vi "OpenCloseThreadWin.vi"(0 "reference in":refnum<class "SuperNS.lvclass">, 2 "Open (F: Close)":bool, 5 "error in":errorcluster) -> (14 "reference out":refnum<class "SuperNS.lvclass">, 19 "error out":errorcluster)   [LabVIEW 2020, in "SuperNS.lvclass"]
doc: "Copyright © 2008 - 2024 VI Technologies B.V. \nALL RIGHTS RESERVED\n\nOpens / Closes the SuperNS's background process frontpanel. This could be usefull for debugging purposes."
uses:
  SuperNS.lvclass
  SuperNS.lvclass/SuperNS.ctl
panel:
  # "Copyright (c) 2024, VI Technologies B.V.\nAll rights reserved.\n\nRedistribution and use in source and binary forms, with or without modification, are permitted provided that \nthe following conditions are met:\n\n * Redistributions of source code must retain the above copyright notice, this list of conditions and the \nfollowing disclaimer.\n * Redistributions in binary form must reproduce the above copyright notice, this list of conditions and the \nfollowing disclaimer in the documentation and/or other materials provided with the distribution.\n * Neither the name of VI Technologies B.V. nor the names of its contributors may be used to endorse or \npromote products derived from this software without specific prior written permission.\n\nTHIS SOFTWARE IS PROVIDED BY THE COPYRIGHT HOLDERS AND CONTRIBUTORS \"AS IS\" AND ANY EXPRESS OR \nIMPLIED WARRANTIES, INCLUDING, BUT NOT LIMITED TO, THE IMPLIED WARRANTIES OF MERCHANTABILITY \nAND FITNESS FOR A PARTICULAR PURPOSE ARE DISCLAIMED. IN NO EVENT SHALL THE COPYRIGHT OWNER OR \nCONTRIBUTORS BE LIABLE FOR ANY DIRECT, INDIRECT, INCIDENTAL, SPECIAL, EXEMPLARY, OR CONSEQUENTIAL \nDAMAGES (INCLUDING, BUT NOT LIMITED TO, PROCUREMENT OF SUBSTITUTE GOODS OR SERVICES; LOSS OF \nUSE, DATA, OR PROFITS; OR BUSINESS INTERRUPTION) HOWEVER CAUSED AND ON ANY THEORY OF LIABILITY, \nWHETHER IN CONTRACT, STRICT LIABILITY, OR TORT (INCLUDING NEGLIGENCE OR OTHERWISE) ARISING IN ANY \nWAY OUT OF THE USE OF THIS SOFTWARE, EVEN IF ADVISED OF THE POSSIBILITY OF SUCH DAMAGE.\n\nFor more information, please visit https://www.vi-tech.nl or contact us at info@vi-tech.nl"
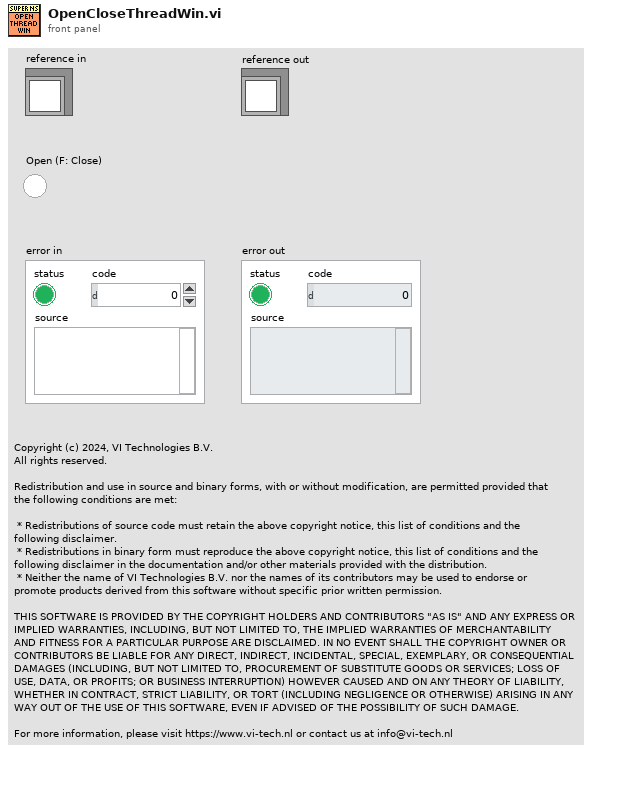
[diagram p1: front panel]
types:
  T1 = typedef "SuperNS.lvclass/ObjectAttributes.ctl" = cluster{"NSName":string, "RemoteEP_URL":string, "BufferSize":i32, "Element Allocation Mode":T2, "ConnLost Timeout":i32, "Writer":bool, "ReadDataEvent":string, "FlushAfterWrite":bool, "Thread":cluster{"VI Refnum":refnum<vi>, "Started Notifier":refnum<notifier>, "Stopped Notifier":refnum<notifier>, "CmdEvent":refnum<user-event>}, "Endpoint":refnum<k21>, "R/W Error":bool, "Flush Wait Condition":T3, "DataReadEvent":refnum<user-event>, "NS Created":bool, "BG ConnCheck/Read period":i32, "ErrorEvent":refnum<user-event>}
  T2 = typedef "Stream Element Allocation Mode.ctl" = u32
  T3 = typedef "Flush And Wait Empty Condition.ctl" = u8
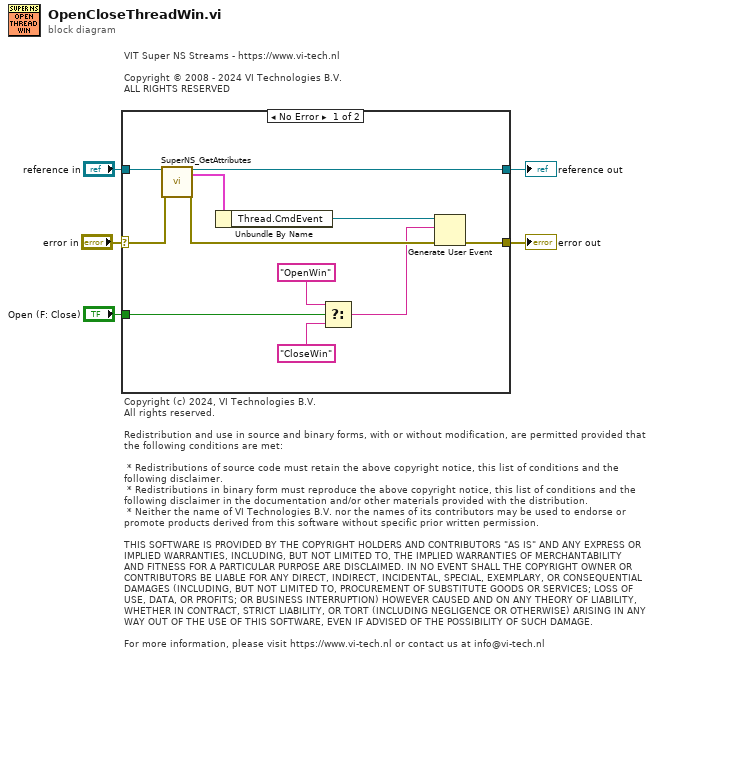
[diagram p0: block diagram]
diagram:
  # "VIT Super NS Streams - https://www.vi-tech.nl\n\nCopyright © 2008 - 2024 VI Technologies B.V. \nALL RIGHTS RESERVED"
  # "Copyright (c) 2024, VI Technologies B.V.\nAll rights reserved.\n\nRedistribution and use in source and binary forms, with or without modification, are permitted provided that \nthe following conditions are met:\n\n * Redistributions of source code must retain the above copyright notice, this list of conditions and the \nfollowing disclaimer.\n * Redistributions in binary form must reproduce the above copyright notice, this list of conditions and the \nfollowing disclaimer in the documentation and/or other materials provided with the distribution.\n * Neither the name of VI Technologies B.V. nor the names of its contributors may be used to endorse or \npromote products derived from this software without specific prior written permission.\n\nTHIS SOFTWARE IS PROVIDED BY THE COPYRIGHT HOLDERS AND CONTRIBUTORS \"AS IS\" AND ANY EXPRESS OR \nIMPLIED WARRANTIES, INCLUDING, BUT NOT LIMITED TO, THE IMPLIED WARRANTIES OF MERCHANTABILITY \nAND FITNESS FOR A PARTICULAR PURPOSE ARE DISCLAIMED. IN NO EVENT SHALL THE COPYRIGHT OWNER OR \nCONTRIBUTORS BE LIABLE FOR ANY DIRECT, INDIRECT, INCIDENTAL, SPECIAL, EXEMPLARY, OR CONSEQUENTIAL \nDAMAGES (INCLUDING, BUT NOT LIMITED TO, PROCUREMENT OF SUBSTITUTE GOODS OR SERVICES; LOSS OF \nUSE, DATA, OR PROFITS; OR BUSINESS INTERRUPTION) HOWEVER CAUSED AND ON ANY THEORY OF LIABILITY, \nWHETHER IN CONTRACT, STRICT LIABILITY, OR TORT (INCLUDING NEGLIGENCE OR OTHERWISE) ARISING IN ANY \nWAY OUT OF THE USE OF THIS SOFTWARE, EVEN IF ADVISED OF THE POSSIBILITY OF SUCH DAMAGE.\n\nFor more information, please visit https://www.vi-tech.nl or contact us at info@vi-tech.nl"
  n1 = case shown="No Error" "error in" {
    selector: "error in" -> [w16 w18]
    tunnel: [w14 w18] -> w1
    tunnel: [w12 w17] -> w4
    tunnel: "reference in" -> [w13 w17]
    tunnel: "Open (F: Close)" -> [w11 _]
    frame No Error {
      n2 = call "SuperNS_GetAttributes.vi"("reference in"=w13, "error in"=w16) -> ("reference out"=w12:refnum<class "SuperNS.lvclass">, "Data"=w7:T1, "error out"=w15:errorcluster)  [unwired: 14 in, 1 out]
      n3 = Unbundle By Name(w7) -> ("Thread.CmdEvent"=w6:refnum<user-event>)
      n4 = Select(t="OpenWin", s=w11, f="CloseWin") -> (s? t:f=w8:string)
      n5 = Generate User Event(user event=w6, event data cluster=w8, error in=w15) -> (error out=w14:errorcluster)  [unwired: 1 in, 1 out]
    }
    frame Error {
    }
  }
  "reference out" <- w4
  "error out" <- w1
